vi "Initialize XML.vi"   [LabVIEW 2016, in "SLL File IO.lvlib"]
doc: "Initialize an XML reference either from an XML file or from an XML string."
uses:
  SLL File IO.lvlib
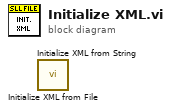
[diagram p0: block diagram]
diagram:
  n1 = call "Initialize XML from File.vi"() -> ()  [unwired: 10 in, 2 out]
  n2 = call "Initialize XML from String.vi"() -> ()  [unwired: 10 in, 2 out]
